vi "Manipulator Jacobian (World Frame).vi"(8 "error in (no error)":errorcluster, 10 "joint positions":dbl[](array[numeric]), 11 "serial arm in":refnum<class "NI_Robotics_Serial Robot Arm.lvclass">) -> (0 "error out":errorcluster, 1 "forward kinematics":T1, 2 "jacobian":T1, 3 "serial arm out":refnum<class "NI_Robotics_Serial Robot Arm.lvclass">)   [LabVIEW 2017, in "NI_Kinematics.lvlib"]
doc: "Generates a Jacobian matrix that transforms differential velocities in joint space to the Cartesian velocity of the end effector in the coordinate frame of the world.\n\n<B>.m file:</B> jacob0"
uses:
  <vilib>/robotics/Kinematics/NI_Kinematics.lvlib
  <vilib>/robotics/Kinematics/Robot/NI_Robotics_Serial Robot Arm.lvclass
  <vilib>/Analysis/Matrix/Datatypes/RealMatrix.ctl
  <vilib>/Analysis/baseanly.llb/Real A x B.vi
  <vilib>/Analysis/NI_AALBase.lvlib
  <vilib>/Analysis/Matrix/NI_Matrix.lvlib
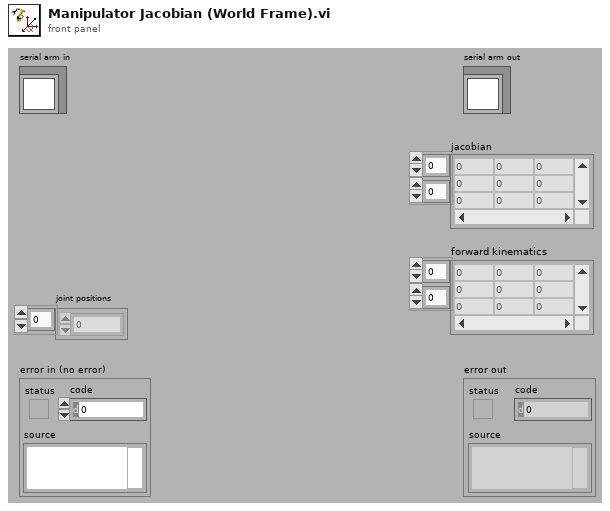
[diagram p1: front panel]
types:
  T1 = typedef "NI_Matrix.lvlib/RealMatrix.ctl" = dbl[][]
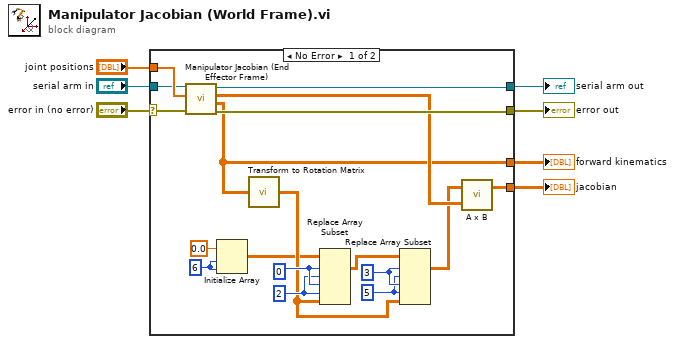
[diagram p0: block diagram]
diagram:
  n1 = case shown="No Error" "error in (no error)" {
    selector: "error in (no error)" -> [w19 w27]
    tunnel: [w23 w27] -> w6
    tunnel: [w24 w26] -> w4
    tunnel: "serial arm in" -> [w20 w26]
    tunnel: "joint positions" -> [w25 _]
    tunnel: [w22 _] -> w2
    tunnel: [w18 _] -> w1
    frame No Error {
      w9 = 6 ("dimension size")
      w13 = 5 ("dimension size")
      w14 = 3 ("dimension size")
      w16 = 2 ("dimension size")
      w17 = 0 ("dimension size")
      n2 = call <vilib>:"Manipulator Jacobian (End Effector Frame).vi"("error in (no error)"=w19, "joint positions"=w25, "serial arm in"=w20) -> ("error out"=w23:errorcluster, "forward kinematics"=w18:T1, "jacobian"=w21:T1, "serial arm out"=w24:refnum<class "NI_Robotics_Serial Robot Arm.lvclass">)  [unwired: 5 out]
      n3 = Initialize Array(0.0 ("element"), w9, w9) -> (w8:dbl[][])
      n4 = call <vilib>:"Transform to Rotation Matrix.vi"("transform"=w18) -> ("rotation matrix"=w12:T1)
      n5 = Replace Array Subset(array=w8, new element=w12, index (dim 0)=w17, index (dim 1)=w16, index (dim 2)=w17, index (dim 3)=w16) -> (w15:T1)
      n6 = Replace Array Subset(array=w15, new element=w12, index (dim 0)=w14, index (dim 1)=w13, index (dim 2)=w14, index (dim 3)=w13) -> (w11:T1)
      n7 = call-poly <vilib>:"A x B.vi"("B"=w21, "A"=w11) -> ("A x B"=w22:T1)  [unwired: 1 out]
    }
    frame Error {
    }
  }
  "error out" <- w6
  "serial arm out" <- w4
  "jacobian" <- w2
  "forward kinematics" <- w1
